vi "pyexample.vi"() -> ()   [LabVIEW 2022 SP3]
uses:
  C:/Program Files (x86)/National Instruments/LabVIEW 2022/examples/Connectivity/Python/support/PythonVersionsEnum.ctl
panel:
  out "return value":dbl
  in  "module path":path
  out "error out":errorcluster
  in  "error in (no error)":errorcluster
  in  "python version":T1
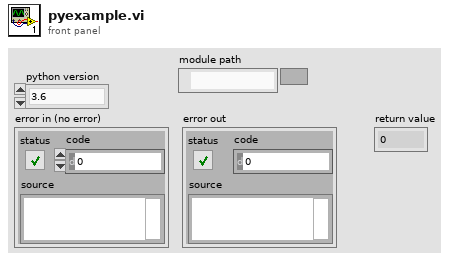
[diagram p1: front panel]
types:
  T1 = typedef "PythonVersionsEnum.ctl" = enum16{"3.6", "3.7", "3.8", "3.9"}
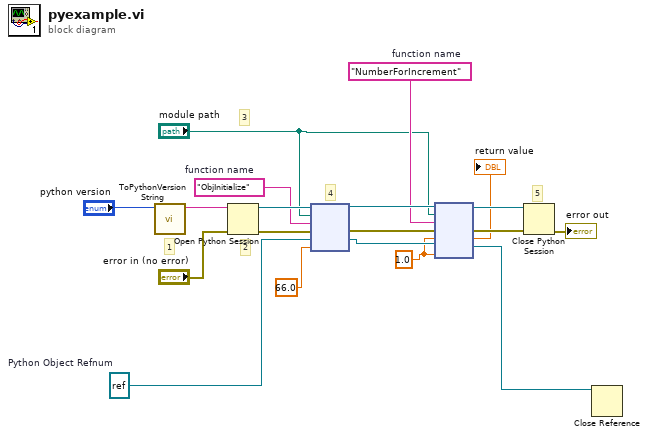
[diagram p0: block diagram]
diagram:
  w2 = "NumberForIncrement"  # function name
  w5 = 1.0
  w12 = refnum<k38> refnum  # Python Object Refnum
  w14 = "ObjInitialize"  # function name
  # "5"
  # "4"
  # "2"
  # "3"
  # "1"
  n1 = call "ToPythonVersionString.vi"("python version"="python version") -> ("python version string"=w19:string)  [unwired: 10 in]
  n2 = Open Python Session(python version=w19, 3:"error in (no error)") -> (session out=w16:refnum<k35>, error out=w15:errorcluster)  [unwired: 1 in]
  n3 = node(w16, "module path", w14, w15, w12, 66.0) -> (w8:refnum<k35>, w11:errorcluster, w7:refnum<k38>)  [unwired: 1 in, 2 out]
  n4 = node(w8, "module path", w2, w11, w5, w7, w5) -> (w9:refnum<k35>, w10:errorcluster, →"return value":dbl, w3:refnum<k38>)  [unwired: 1 in, 2 out]
  n5 = Close Python Session(session in=w9, error in=w10) -> (11:→"error out":errorcluster)
  n6 = Close Reference(reference=w3) -> ()  [unwired: 1 in, 1 out]
